vi "电信1801-2018012704-杜兴安-虚拟仪器作业1.vi"() -> ()   [LabVIEW 2020]
panel:
  out "数组 2":dbl[][](array[numeric])
  out "输出数组 2":dbl[][](array[numeric])
  in  "输入数组 2":dbl[][](array[numeric])
  in  "替换的行号":dbl
  in  "替换数组":dbl[](array[numeric])
  out "输出数组":dbl[][](array[numeric])
  in  "输入数组":dbl[][](array[numeric])
  out "删除部分":dbl[][](array[numeric])
  out "输出数组":dbl[][](array[numeric])
  in  "输入数组":dbl[][](array[numeric])
  in  "插入的行号":dbl
  in  "插入的子数组":dbl[](array[numeric])
  out "输出数组":dbl[][](array[numeric])
  in  "输入数组":dbl[][](array[numeric])
  in  "列数":dbl
  in  "行数":dbl
  in  "列数":dbl
  in  "行数":dbl
  out "?":dbl[](array[numeric])
  out "?":dbl[](array[numeric])
  out "?":dbl
  in  "数组":dbl[][](array[numeric])
  out "二维数组长度":dbl[](array[numeric])
  out "一维数组长度":dbl
  in  "二维数组":dbl[][](array[numeric])
  in  "一维数组":dbl[](array[numeric])
  # "2"
  # "1"
  # "3"
  # "4"
  # "5"
  # "6"
  # "7"
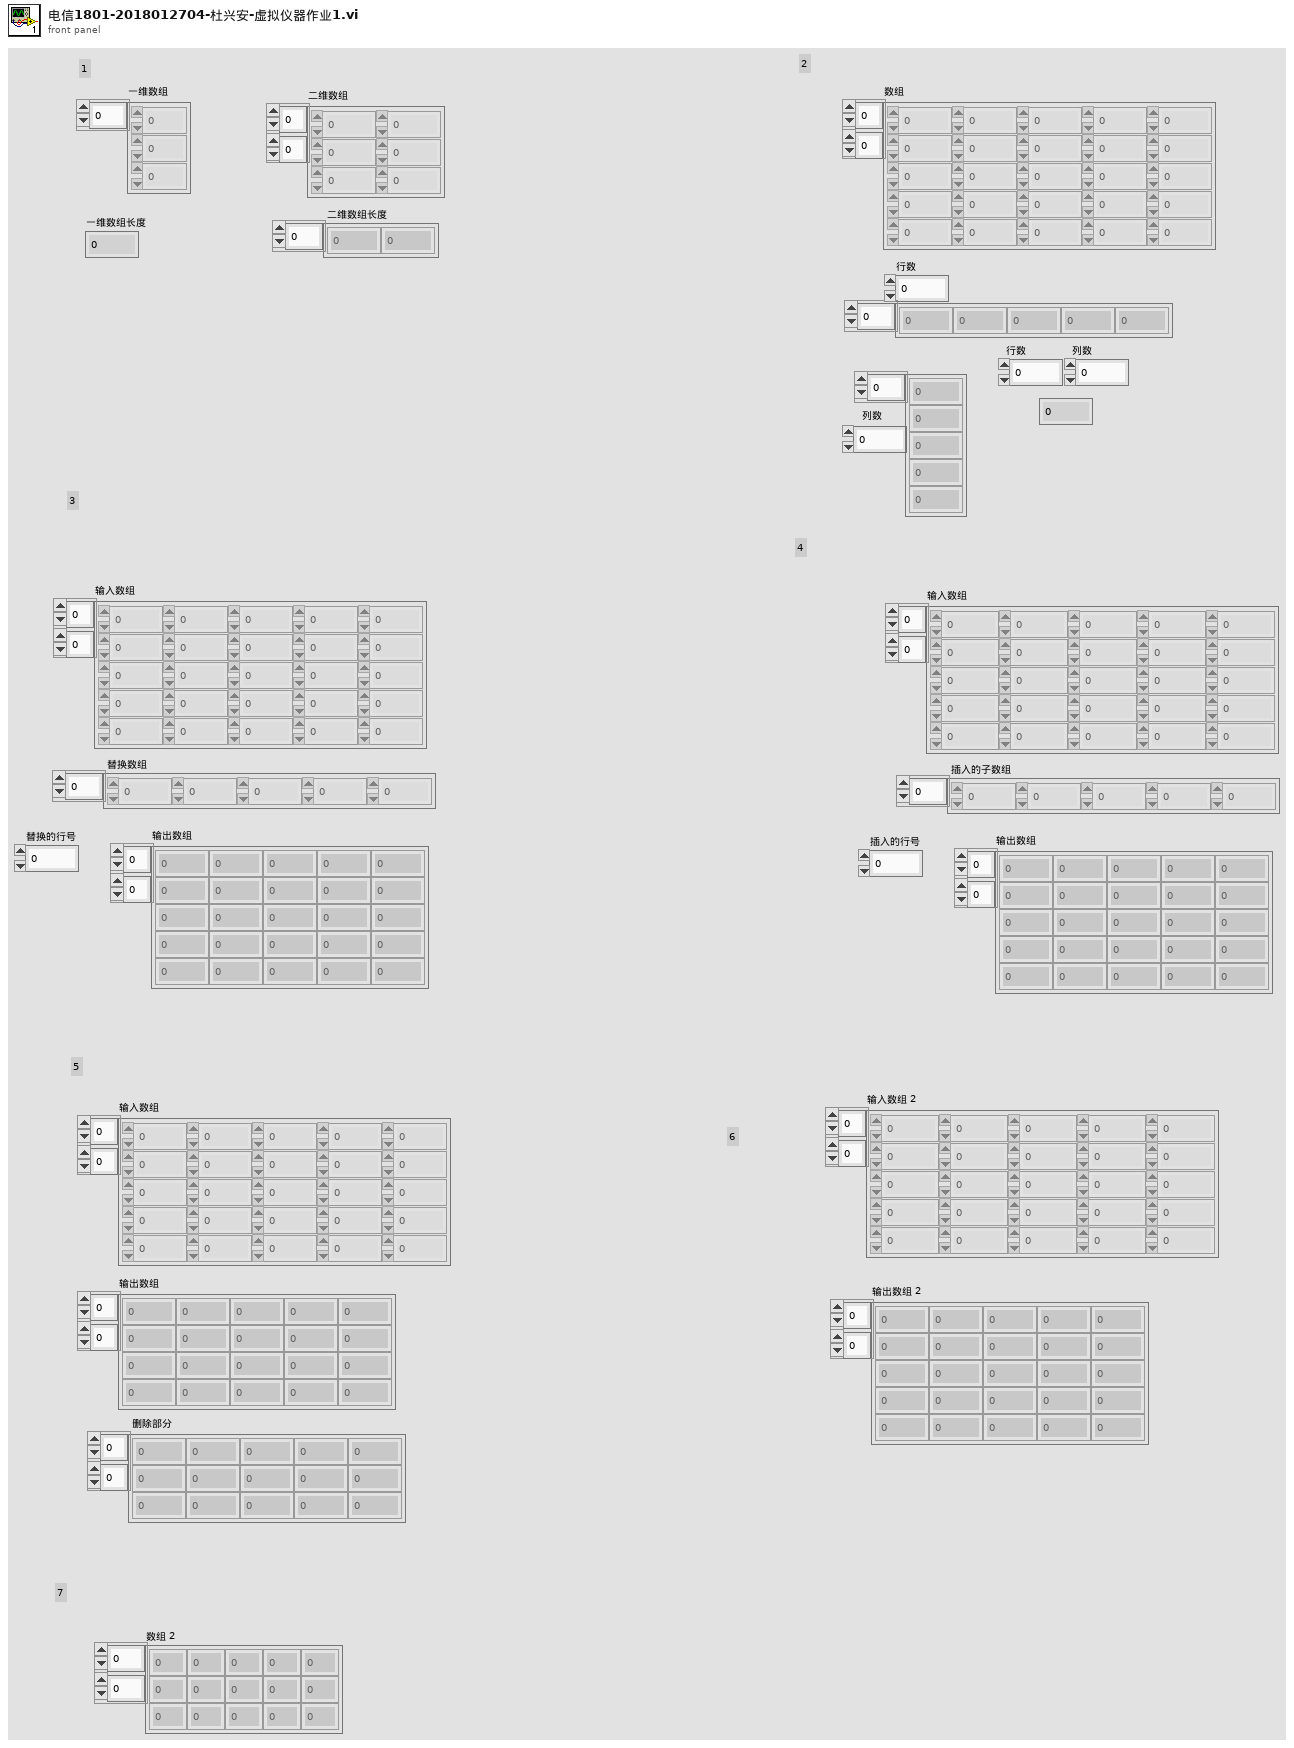
[diagram p1: front panel]
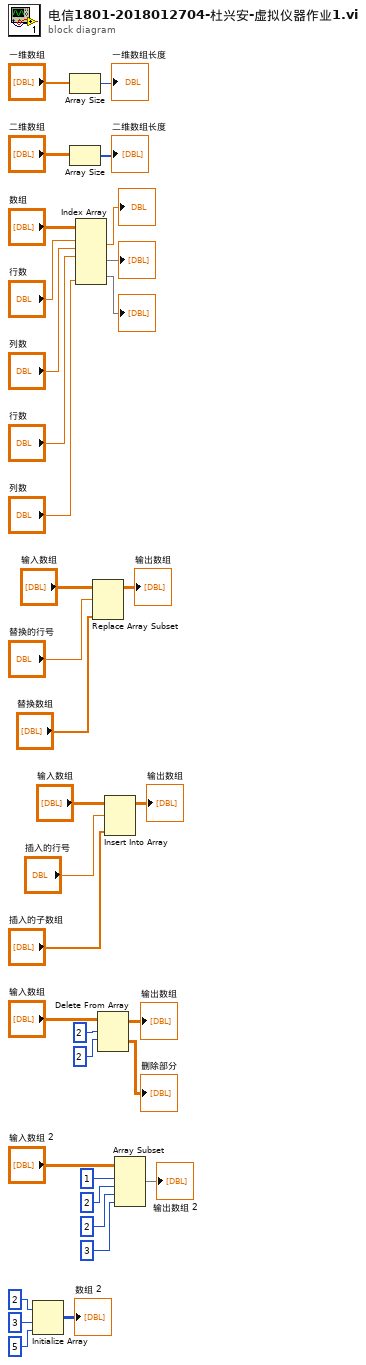
[diagram p0: block diagram]
diagram:
  n1 = Initialize Array(2, 3, 5) -> (→"数组 2":i32[][])
  n2 = Array Size(array="一维数组") -> (size(s)=→"一维数组长度":i32)
  n3 = Array Size(array="二维数组") -> (size(s)=→"二维数组长度":i32[])
  n4 = Index Array(array="数组", index (row) #1="行数", index (col) #1="列数", index (row) #2="行数", index (col) #3="列数") -> (element #1=→"?":dbl, element #2=→"?":dbl[], element #3=→"?":dbl[])  [unwired: 2 in]
  n5 = Replace Array Subset(array="输入数组", new element="替换数组", index (row)="替换的行号") -> (→"输出数组":dbl[][])  [unwired: 1 in]
  n6 = Delete From Array(array="输入数组", length=2, index (row)=2) -> (deleted portion=→"删除部分":dbl[][], array with subset deleted=→"输出数组":dbl[][])  [unwired: 1 in]
  n7 = Insert Into Array(array="输入数组", index (row)="插入的行号", new element="插入的子数组") -> (→"输出数组":dbl[][])  [unwired: 1 in]
  n8 = Array Subset(array="输入数组 2", index (row)=1, length (row)=2, index (col)=2, length (col)=3) -> (→"输出数组 2":dbl[][])
